vi "Enqueue Message (Array).vi"(8 "Error In":errorcluster, 9 "Message Positions":T2[](array[typedef]), 10 "Data":variant[](array[variant]), 11 "State Machine Messages":T1[](array[typedef])) -> (0 "Error Out":errorcluster)   [LabVIEW 2023, in "QSM - IODocs.lvlib"]
doc: "This VI enqueues an array of messages in the message queue at the specified positions for the Queued State Machine template."
uses:
  QSM - IODocs.lvlib
  Controls/Message Queue Element Position.ctl
  Controls/State Machine Message.ctl
  Controls/Message Queue Reference Functional Global Variable Operation.ctl
  Controls/Message Queue Element.ctl
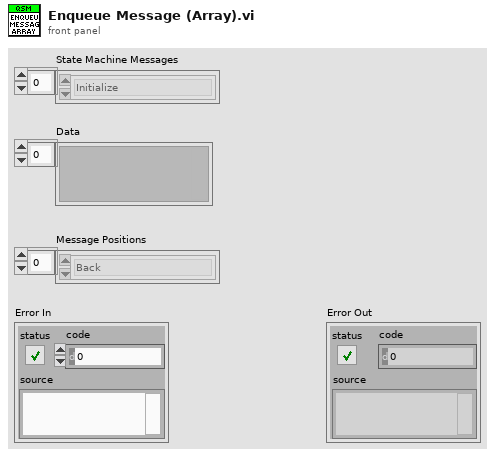
[diagram p1: front panel]
types:
  T1 = typedef "QSM - IODocs.lvlib/State Machine Message.ctl" = enum16{"Initialize", "Handle Error", "Exit"}
  T2 = typedef "QSM - IODocs.lvlib/Message Queue Element Position.ctl" = enum16{"Front", "Back"}
  T3 = typedef "QSM - IODocs.lvlib/Message Queue Reference Functional Global Variable Operation.ctl" = enum16{"Set", "Get"}
  T4 = typedef "QSM - Library.lvlib/Message Queue Reference.ctl" = refnum<queue>
  T5 = typedef "QSM - IODocs.lvlib/Message Queue Element.ctl" = cluster{"State Machine Message":T1, "Data":variant}
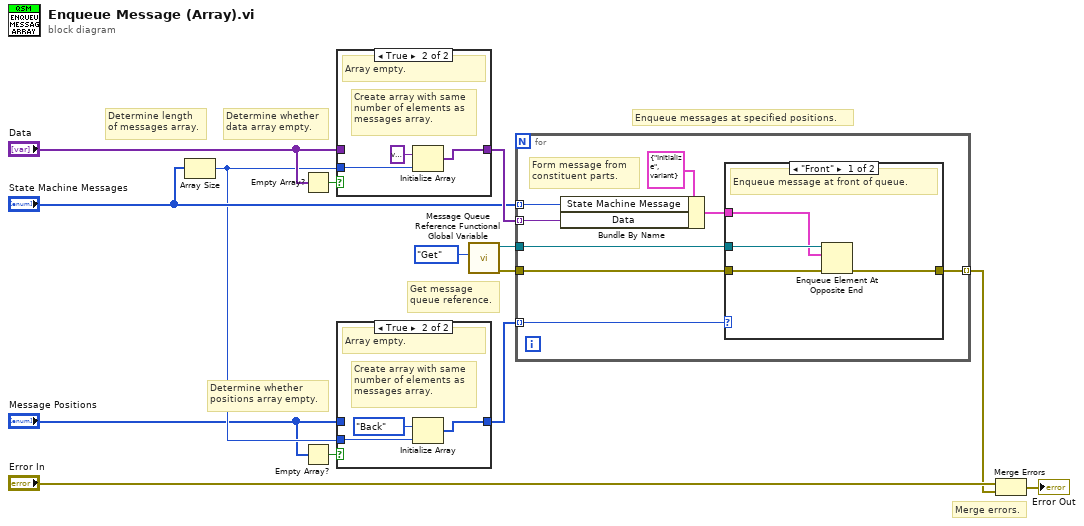
[diagram p0: block diagram]
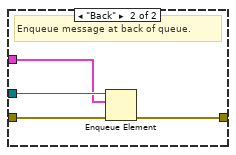
[diagram p4: hidden frame]
diagram:
  # "Merge errors."
  # "Determine whether\npositions array empty."
  # "Determine length\nof messages array."
  # "Determine whether\ndata array empty."
  # "Get message\nqueue reference."
  # "Enqueue messages at specified positions."
  n1 = Array Size(array="State Machine Messages") -> (size(s)=w6:i32)
  n2 = Empty Array?(array="Data") -> (empty?=w11:bool)
  n3 = Empty Array?(array="Message Positions") -> (empty?=w7:bool)
  n4 = case shown="True" w11 {
    tunnel: "Data" -> [w15 _]
    tunnel: [w15 w16] -> w9
    tunnel: w6 -> [_ w18]
    frame False {
      # "Array not empty."
    }
    frame True {
      # "Create array with same\nnumber of elements as\nmessages array."
      # "Array empty."
      n5 = Initialize Array(variant, w18) -> (w16:variant[])
    }
  }
  n6 = case shown="True" w7 {
    tunnel: "Message Positions" -> [w19 _]
    tunnel: [w19 w21] -> w4
    tunnel: w6 -> [_ w22]
    frame False {
      # "Array not empty."
    }
    frame True {
      # "Create array with same\nnumber of elements as\nmessages array."
      # "Array empty."
      n7 = Initialize Array(Message_Queue_Element_Position."Back" ("Message Position"), w22) -> (w21:T2[])
    }
  }
  n8 = call "Message Queue Reference Functional Global Variable.vi"("Operation"=Message_Queue_Reference_Functional_Global_Variable_Operation."Get") -> ("Error Out"=w14:errorcluster, "Message Queue Reference Out"=w13:T4)  [unwired: 9 in]
  n9 = for {
    tunnel: w13 -> [w28]
    tunnel: w4 -> [w27] mode=indexing
    tunnel: "State Machine Messages" -> [w24] mode=indexing
    tunnel: w9 -> [w23] mode=indexing
    tunnel: w14 -> [w30]
    tunnel: [w29] -> w1 mode=indexing
    # "Form message from\nconstituent parts."
    n10 = Bundle By Name(cluster=T5 {"State Machine Message"=enum."Initialize", "Data"=variant} ("Message Queue Element"), "State Machine Message"=w24, "Data"=w23) -> (w25:T5)
    n11 = case shown="\"Front\"" w27 {
      tunnel: w30 -> [w34 w38]
      tunnel: [w33 w37] -> w29
      tunnel: w28 -> [w32 w36]
      tunnel: w25 -> [w31 w35]
      frame "Front" {
        # "Enqueue message at front of queue."
        n12 = Enqueue Element At Opposite End(queue=w32, element=w31, error in (no error)=w34) -> (error out=w33:errorcluster)  [unwired: 1 in, 2 out]
      }
      frame "Back" {
        # "Enqueue message at back of queue."
        n13 = Enqueue Element(queue=w36, element=w35, error in (no error)=w38) -> (error out=w37:errorcluster)  [unwired: 1 in, 2 out]
      }
    }
  }
  n14 = Merge Errors("Error In", w1) -> (→"Error Out":errorcluster)
